vi "Ex5-write-data.vi"() -> ()   [LabVIEW 2021]
uses:
  <vilib>/Utility/NIReport.llb/Report Type.ctl
  <vilib>/addons/_office/excel.llb/Excel Get Data ([dbl]).vi
  <vilib>/addons/_office/excel.llb/Excel Easy Table (str).vi
  <vilib>/addons/_office/excel.llb/Excel Easy Table (num).vi
  <vilib>/Utility/NIReport.llb/NI_report.lvclass
  <vilib>/Utility/NIReport.llb/NI_ReportGenerationCore.lvlib
  <vilib>/Utility/NIReport.llb/Excel/NI_Excel.lvclass
  <vilib>/addons/_office/NI_ReportGenerationToolkit.lvlib
panel:
  in  "outside border":T1={"on/off"=FALSE, "weight"=2, "color"=0} {"weight" items=["xlHairline"=1, "xlMedium"=-4138, "xlThick"=4, "xlThin"=2]}
  in  "inside border":T1={"on/off"=FALSE, "weight"=2, "color"=0} {"weight" items=["xlHairline"=1, "xlMedium"=-4138, "xlThick"=4, "xlThin"=2]}
  in  "Save Button":bool
  in  "Write data":dbl[][](array[numeric]) format="%.2f"
  out "get data":dbl[][](array[numeric]) format="%.2f"
  out "size(s)":i32[](array[numeric])
  in  "stop":bool
  out "MS Office parameters out":T2
  in  "Text Ring":u16(ring) items=["data1", "data2", "data3", "data4", "data5", "summary"]
  out "Work sheet names":string[](array[string])
  out "Count":i32
  in  "file path (use dialog)":path
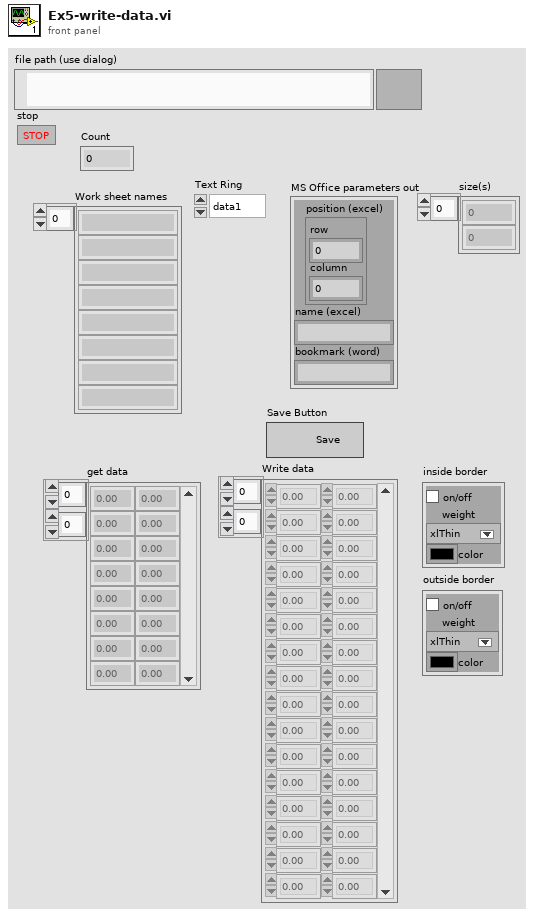
[diagram p1: front panel]
types:
  T1 = cluster{"on/off":bool, "weight":i32, "color":u32}
  T2 = cluster{"position (excel)":cluster{"row":i32, "column":i32}, "name (excel)":string, "bookmark (word)":string}
  T3 = enum16{"open", "replace", "create", "open or create", "replace or create", "replace or create with confirmation"}
  T4 = typedef "NI_ReportGenerationCore.lvlib/Report Type.ctl" = enum16{"HTML", "Word", "Excel"}
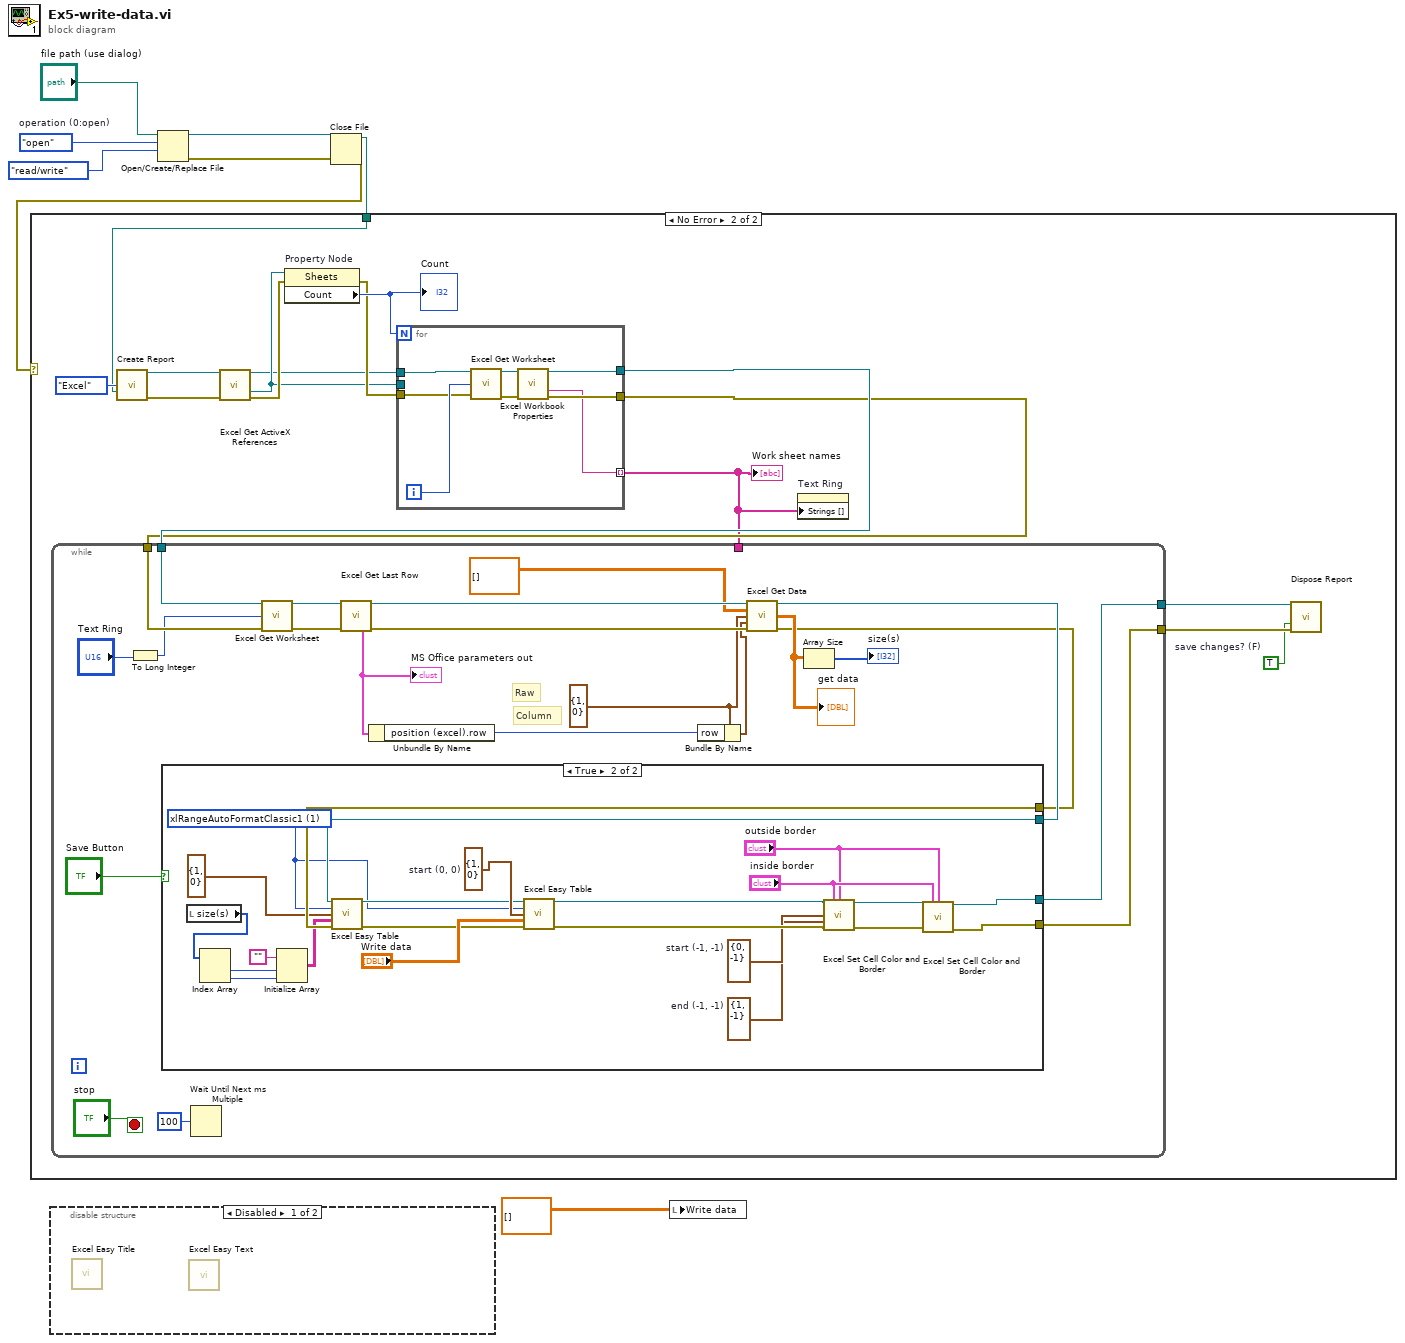
[diagram p0: block diagram]
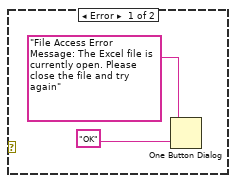
[diagram p3: hidden frame]
diagram:
  w5 = T3."open"  # operation (0:open)
  n1 = disable-structure shown="Disabled" {
    frame Disabled {
      n2 = call <vilib>:"Excel Easy Title.vi"() -> ()  [unwired: 13 in, 3 out]
      n3 = call <vilib>:"Excel Easy Text.vi"() -> ()  [unwired: 11 in, 5 out]
    }
    frame Enabled {
    }
  }
  n4 = Open/Create/Replace File(file path (use dialog)="file path (use dialog)", operation (0:open)=w5, access (0:read/write)=enum16{"read/write", "read-only", "write-only"}."read/write") -> (refnum out=w8:refnum<file>, error out=w7:errorcluster)  [unwired: 3 in, 1 out]
  n5 = Close File(refnum=w8, error in=w7) -> (path=w2:path, error out=w3:errorcluster)
  n6 = case shown="No Error" w3 {
    tunnel: w2 -> [_ w24]
    frame Error {
      n7 = One Button Dialog(message="File Access Error Message: The Excel file is currently open. Please close the file and try again", button name ("OK")="OK") -> ()  [unwired: 1 out]
    }
    frame No Error {
      w11 = TRUE  # save changes? (F)
      n8 = call <vilib>:"Create Report.vi"("report type"=Report_Type."Excel", "template (empty)"=w24) -> ("report out"=w23:refnum<class "NI_report.lvclass">, "error out"=w22:errorcluster)  [unwired: 12 in]
      n9 = call <vilib>:"Excel Get ActiveX References.vi"("report in"=w23, "error in (no error)"=w22) -> ("report out"=w17:refnum<class "NI_report.lvclass">, "Excel.Sheets"=w18:refnum<k7>, "error out"=w20:errorcluster)  [unwired: 7 in, 4 out]
      n10 = property on="Property Node" class="Sheets"(reference=w18, error in=w20) -> (error out=w19:errorcluster, "Count"=w21:i32)  [unwired: 1 out]
      "Count" <- w21
      n11 = for {
        N: w21 -> [_]
        tunnel: w19 -> [w74]
        tunnel: w18 -> [_]
        tunnel: w17 -> [w79]
        tunnel: [w77] -> w16
        tunnel: [w75] -> w15
        tunnel: [w73] -> w14 mode=indexing
        i -> [w80]
        n12 = call <vilib>:"Excel Get Worksheet.vi"("report in"=w79, "worksheet index (0)"=w80, "error in (no error)"=w74) -> ("report out"=w78:refnum<class "NI_report.lvclass">, "error out"=w76:errorcluster)  [unwired: 11 in]
        n13 = call <vilib>:"Excel Workbook Properties.vi"("report in"=w78, "error in (no error)"=w76) -> ("report out"=w77:refnum<class "NI_report.lvclass">, "current worksheet name"=w73:string, "error out"=w75:errorcluster)  [unwired: 10 in, 1 out]
      }
      "Work sheet names" <- w14
      n14 = while {
        tunnel: w14 -> [_]
        tunnel: w16 -> [w47]
        tunnel: w15 -> [w46]
        tunnel: [w28] -> w13
        tunnel: [w27] -> w12
        stop <- "stop" stop-if-true
        w34 = cluster{"row":i32, "column":i32} {"row"=1, "column"=0} ("start (-1, -1)")
        # "Raw"
        # "Column"
        n15 = To Long Integer(number="Text Ring") -> (32bit integer=w44:i32)
        n16 = Wait Until Next ms Multiple(millisecond multiple=u32 100) -> ()  [unwired: 1 out]
        n17 = call <vilib>:"Excel Get Worksheet.vi"("report in"=w47, "worksheet index (0)"=w44, "error in (no error)"=w46) -> ("report out"=w43:refnum<class "NI_report.lvclass">, "error out"=w42:errorcluster)  [unwired: 11 in]
        n18 = call <vilib>:"Excel Get Last Row.vi"("report in"=w43, "error in (no error)"=w42) -> ("report out"=w39:refnum<class "NI_report.lvclass">, "MS Office parameters out"=w33:T2, "error out"=w37:errorcluster)  [unwired: 11 in]
        "MS Office parameters out" <- w33
        n19 = Unbundle By Name(w33) -> ("position (excel).row"=w32:i32)
        n20 = Bundle By Name(cluster=w34, "row"=w32) -> (w31:cluster{"row":i32, "column":i32})
        n21 = call-poly <vilib>:"Excel Get Data.vi"("report in"=w39, "data type"=dbl[][] [], "start (-1, -1)"=w34, "end (-1, -1)"=w31, "error in (no error)"=w37) -> ("report out"=w30:refnum<class "NI_report.lvclass">, "data"=w36:dbl[][], "error out"=w29:errorcluster)  [unwired: 8 in]
        "get data" <- w36
        n22 = case shown="True" "Save Button" {
          tunnel: w30 -> [w48 w68]
          tunnel: w29 -> [w49 w67]
          tunnel: [w48 w53] -> w28
          tunnel: [w49 w52] -> w27
          frame False {
          }
          frame True {
            w56 = 1 items=["xlRangeAutoFormat3DEffects1"=13, "xlRangeAutoFormat3DEffects2"=14, "xlRangeAutoFormatAccounting1"=4, "xlRangeAutoFormatAccounting2"=5, "xlRangeAutoFormatAccounting3"=6, "xlRangeAutoFormatAccounting4"=17, "xlRangeAutoFormatClassic1"=1, "xlRangeAutoFormatClassic2"=2, "xlRangeAutoFormatClassic3"=3, "xlRangeAutoFormatColor1"=7, "xlRangeAutoFormatColor2"=8, "xlRangeAutoFormatColor3"=9, "xlRangeAutoFormatList1"=10, "xlRangeAutoFormatList2"=11, "xlRangeAutoFormatList3"=12, "xlRangeAutoFormatLocalFormat1"=15, "xlRangeAutoFormatLocalFormat2"=16, "xlRangeAutoFormatLocalFormat3"=19, "xlRangeAutoFormatLocalFormat4"=20, "xlRangeAutoFormatReport1"=21, "xlRangeAutoFormatReport2"=22, "xlRangeAutoFormatReport3"=23, "xlRangeAutoFormatReport4"=24, "xlRangeAutoFormatReport5"=25, "xlRangeAutoFormatReport6"=26, "xlRangeAutoFormatReport7"=27, "xlRangeAutoFormatReport8"=28, "xlRangeAutoFormatReport9"=29, "xlRangeAutoFormatReport10"=30, "xlRangeAutoFormatClassicPivotTable"=31, "xlRangeAutoFormatTable1"=32, "xlRangeAutoFormatTable2"=33, "xlRangeAutoFormatTable3"=34, "xlRangeAutoFormatTable4"=35, "xlRangeAutoFormatTable5"=36, "xlRangeAutoFormatTable6"=37, "xlRangeAutoFormatTable7"=38, "xlRangeAutoFormatTable8"=39, "xlRangeAutoFormatTable9"=40, "xlRangeAutoFormatTable10"=41, "xlRangeAutoFormatPTNone"=42, "xlRangeAutoFormatNone"=-4142, "xlRangeAutoFormatSimple"=-4154] ("auto format (none)")
            w57 = cluster{"row":i32, "column":i32} {"row"=1, "column"=-1}  # end (-1, -1)
            w58 = cluster{"row":i32, "column":i32} {"row"=0, "column"=-1}  # start (-1, -1)
            w71 = cluster{"row":i32, "column":i32} {"row"=1, "column"=0}  # start (0, 0)
            n23 = local read "size(s)"() -> (w65:i32[])
            n24 = Index Array(array=w65) -> (element #1=w64:i32, element #2=w63:i32)  [unwired: 2 in]
            n25 = Initialize Array("", w64, w63) -> (w62:string[][])
            n26 = call-poly <vilib>:"Excel Easy Table.vi"("report in"=w68, "auto format (none)"=w56, "start (0, 0)"=cluster{"row":i32, "column":i32} {"row"=1, "column"=0}, "text data"=w62, "error in (no error)"=w67) -> ("report out"=w70:refnum<class "NI_report.lvclass">, "error out"=w69:errorcluster)  [unwired: 6 in, 3 out]
            n27 = call-poly <vilib>:"Excel Easy Table.vi"("report in"=w70, "auto format (none)"=w56, "start (0, 0)"=w71, "text data"="Write data", "error in (no error)"=w69) -> ("report out"=w60:refnum<class "NI_report.lvclass">, "error out"=w59:errorcluster)  [unwired: 6 in, 3 out]
            n28 = call <vilib>:"Excel Set Cell Color and Border.vi"("report in"=w60, "inside border"="inside border", "outside border"="outside border", "start (-1, -1)"=w58, "end (-1, -1)"=w57, "error in (no error)"=w59) -> ("report out"=w55:refnum<class "NI_report.lvclass">, "error out"=w54:errorcluster)  [unwired: 8 in]
            n29 = call <vilib>:"Excel Set Cell Color and Border.vi"("report in"=w55, "inside border"="inside border", "outside border"="outside border", "error in (no error)"=w54) -> ("report out"=w53:refnum<class "NI_report.lvclass">, "error out"=w52:errorcluster)  [unwired: 10 in]
          }
        }
        n30 = Array Size(array=w36) -> (size(s)=→"size(s)":i32[])
      }
      n31 = property on="Text Ring" class="Ring (strict)"("Strings []"=w14) -> ()  [unwired: 2 in, 2 out]
      n32 = call-dynamic "Dispose Report.vi"("report in"=w13, "save changes? (F)"=w11, "error in (no error)"=w12) -> ()  [unwired: 12 in, 1 out]
    }
  }
  n33 = local write "Write data"(dbl[][] [] ("Write data")) -> ()
